vi "Write Control Refnum.vi"(10 "Ctl Refnum":refnum<vi>, 11 "TerminalReference in":refnum<class "TerminalPropertyBinding.lvclass">) -> (3 "TerminalReferenceBinding Out":refnum<class "TerminalPropertyBinding.lvclass">)   [LabVIEW 2017, in "TerminalPropertyBinding.lvclass"]
doc: "<License>\nCopyright © 2017 Composed Systems, LLC | All rights reserved\nwww.composed.io\n\nAuthor: Ethan Stern <ethan.stern@composed.io>\n\nThis software is provided \"AS IS\" WITHOUT WARRANTIES, either express or implied, AND IS FOR EDUCATIONAL PURPOSES ONLY.\n</License>"
uses:
  <vilib>/gpm_packages/@cs/transport/Source/Concrete/TerminalPropertyBinding/TerminalPropertyBinding.lvclass
  <vilib>/gpm_packages/@cs/transport/Source/Concrete/TerminalPropertyBinding/TerminalPropertyBinding.lvclass/TerminalPropertyBinding.ctl
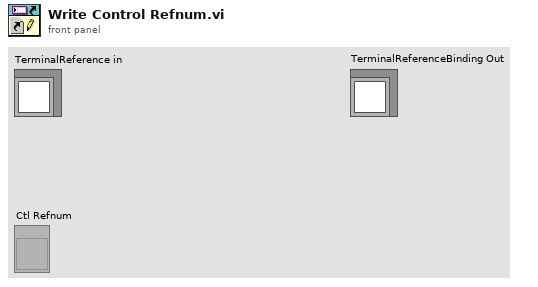
[diagram p1: front panel]
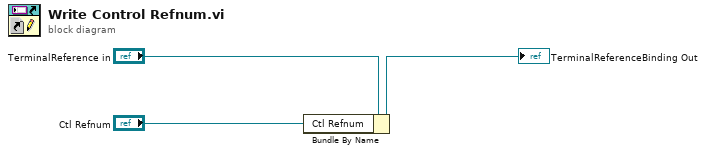
[diagram p0: block diagram]
diagram:
  n1 = Bundle By Name(cluster="TerminalReference in", "Ctl Refnum"="Ctl Refnum") -> (→"TerminalReferenceBinding Out":refnum<class "TerminalPropertyBinding.lvclass">)
